vi "PathPlanner_ObstacleGrid_ProcessNavFile.vi"(11 "PathPlanner_Grid":T2) -> (3 "NavGridObstacles":T1[](array[typedef]))   [LabVIEW 2019, in "PathPlanner24.lvlib"]
doc: "Load an obstacle grid from a JSON formatted file. \n\nInputs: \n - filename - string - The name of the obstacle grid file. See notes below on file naming.\n\nOutputs:\n - PathPlanner_ObstacleGrid - cluster - Obstacle grid read from JSON file.\n - Error out - cluster - Error cluster\n - Full Filename - string - fully qualified file name.\n\nNotes on file naming:\n - The file name must include the extention. \".json\" is not automatically appended to the name. \n - The file name can be a simple file or an absolute path. If a simple file name is used the default path on the RoboRIO is: \"home:\\lvuser\\natinst\\LabVIEW Data\". On a Windows PC the default path is the LabVIEW default directory. Normally this is: “%HOMEDRIVE%%HOMEPATH%\\Documents\\LabView Data\".\n - Filenames on the RoboRIO, which runs Linux, are case sensitive."
uses:
  PathPlanner24.lvlib
  TypeDef/PathPlannerObstacleGrid.ctl
  TypeDef/PathPlannerFinderGridPosition.ctl
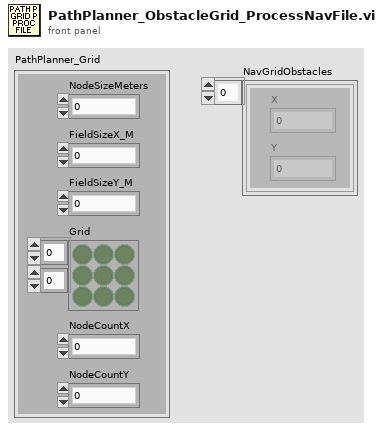
[diagram p1: front panel]
types:
  T1 = typedef "PathPlanner24.lvlib/PathPlannerFinderGridPosition.ctl" = cluster{"X":i32, "Y":i32}
  T2 = typedef "PathPlanner24.lvlib/PathPlannerObstacleGrid.ctl" = cluster{"NodeSizeMeters":dbl, "Grid":bool[][], "NodeCountX":i32, "NodeCountY":i32, "FieldSizeX_M":dbl, "FieldSizeY_M":dbl}
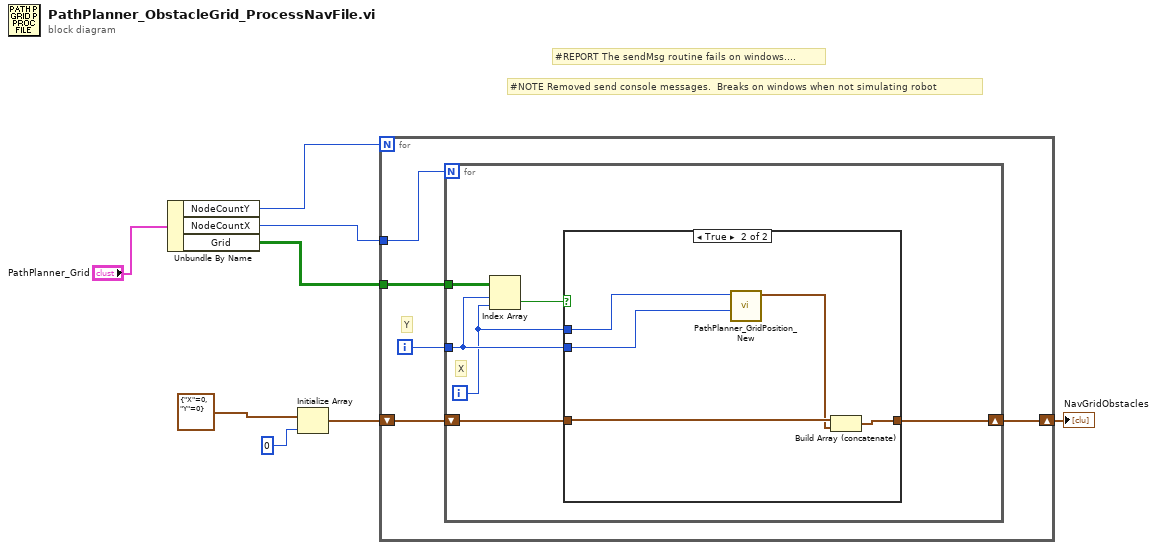
[diagram p0: block diagram]
diagram:
  # "#NOTE Removed send console messages.  Breaks on windows when not simulating robot"
  # "#REPORT The sendMsg routine fails on windows...."
  n1 = Unbundle By Name("PathPlanner_Grid") -> ("NodeCountY"=w7:i32, "NodeCountX"=w6:i32, "Grid"=w5:bool[][])
  n2 = Initialize Array(T1 {"X"=0, "Y"=0} ("PathPlannerFinderGridPosition"), 0 ("dimension size")) -> (w2:T1[])
  n3 = for {
    N: w7 -> [_]
    tunnel: w6 -> [w13]
    tunnel: w5 -> [w12]
    shift-right: [w9] -> w1
    shift-left: w2 -> [w10]
    i -> [w11]
    # "Y"
    n4 = for {
      N: w13 -> [_]
      tunnel: w12 -> [w19]
      tunnel: w11 -> [w15]
      shift-right: [w16] -> w9
      shift-left: w10 -> [w17]
      i -> [w14]
      # "X"
      n5 = Index Array(array=w19, index (row)=w15, index (col)=w14) -> (element=w18:bool)
      n6 = case shown="True" w18 {
        tunnel: w17 -> [w20 w25]
        tunnel: [w20 w24] -> w16
        tunnel: w15 -> [_ w21]
        tunnel: w14 -> [_ w22]
        frame False {
        }
        frame True {
          n7 = call "PathPlanner_GridPosition_New.vi"("Int Y"=w21, "Int X"=w22) -> ("GridPosition"=w23:T1)  [unwired: 9 in]
          n8 = Build Array (concatenate)(w25, w23) -> (w24:T1[])
        }
      }
    }
  }
  "NavGridObstacles" <- w1
